vi "circular buffer test.vi"() -> ()   [LabVIEW 2010]
panel:
  out "size(s) 4":i32
  out "size(s) 3":i32
  out "size(s) 2":i32
  in  "stop":bool
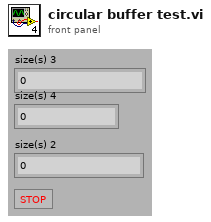
[diagram p1: front panel]
types:
  T1 = enum16{"CreateBuffer", "WriteBytes", "WriteByte", "AvailableMemory", "OccupiedMemory", "CheckBytes", "ReadBytes"}
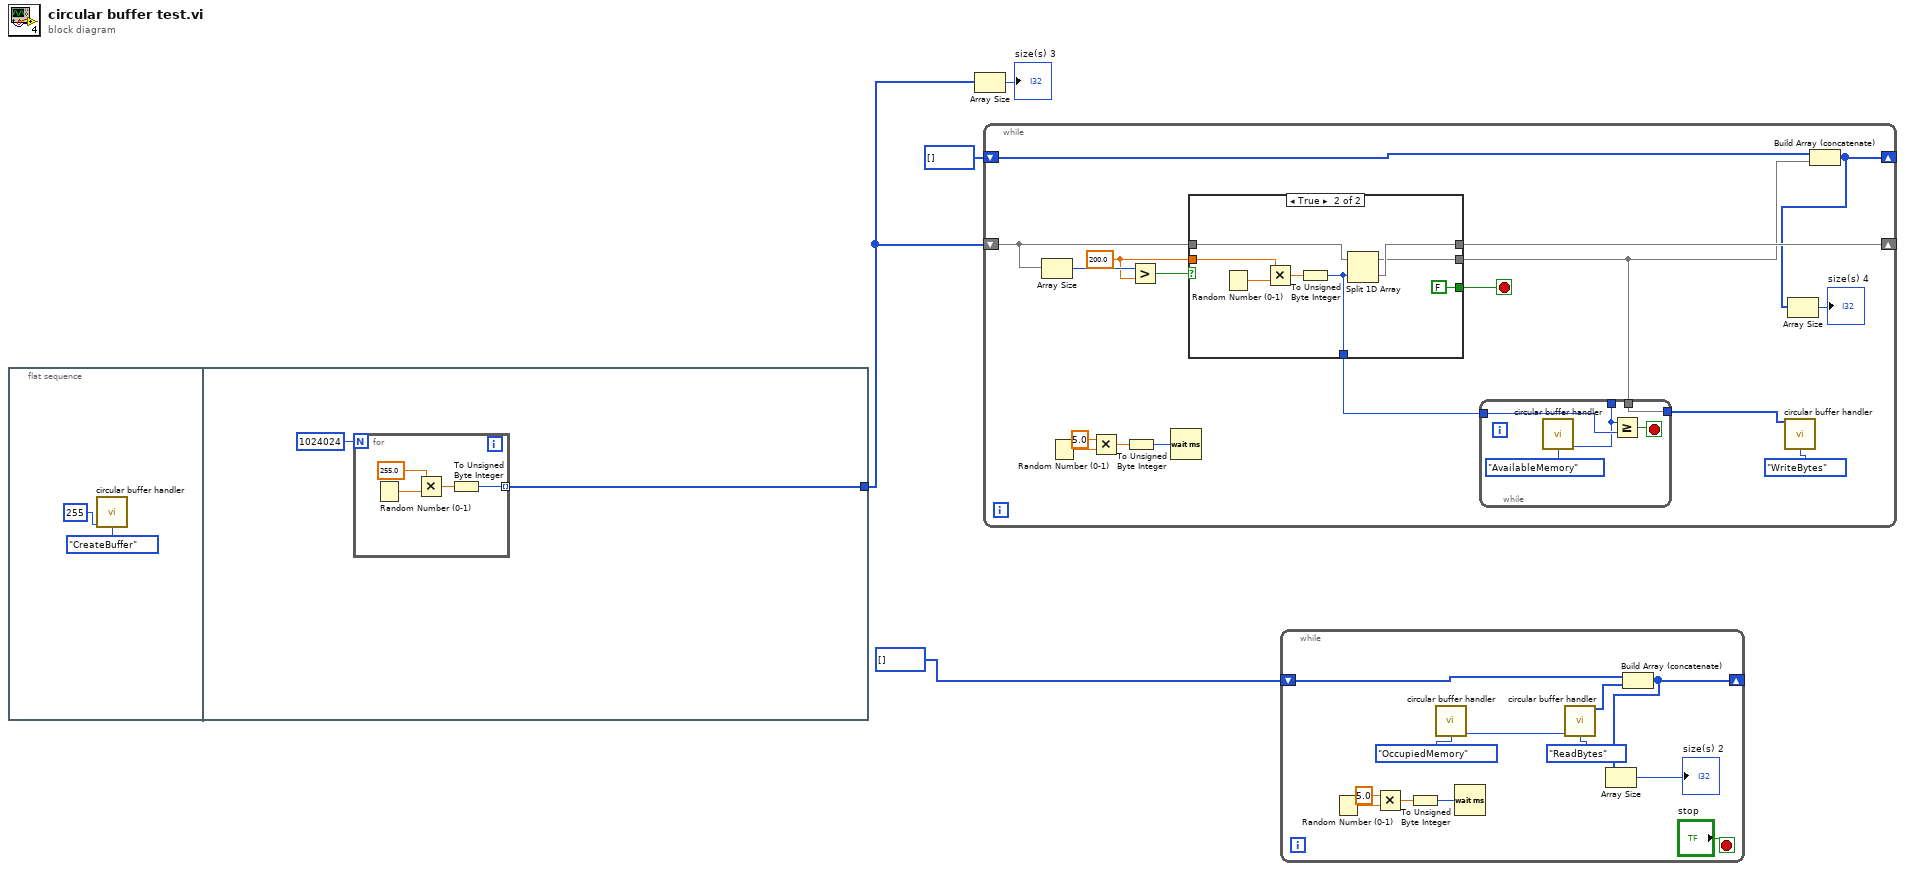
[diagram p0: block diagram]
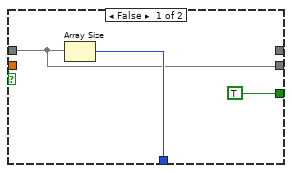
[diagram p2: hidden frame]
diagram:
  n1 = flat-sequence {
    tunnel: [w7] -> w2
    frame #0 {
      n2 = call "circular buffer handler.vi"("NumberOfBytes"=255 ("ByteToWrite"), "Enum"=T1."CreateBuffer") -> ()  [unwired: 11 in, 3 out]
    }
    frame #1 {
      n3 = for {
        N: 1024024 -> [_]
        tunnel: [w9] -> w7 mode=indexing
        n4 = Random Number (0-1)() -> (number: 0 to 1=w12:dbl)
        n5 = Multiply(x=255.0, y=w12) -> (x*y=w10:dbl)
        n6 = To Unsigned Byte Integer(number=w10) -> (unsigned 8bit integer=w9:u8)
      }
    }
  }
  n7 = Array Size(array=w2) -> (size(s)=→"size(s) 3":i32)
  n8 = while {
    shift-right: [w28] -> _
    shift-left: w2 -> [w26]
    shift-right: [w13] -> _
    shift-left: u8[] [] -> [w21]
    stop <- w22 stop-if-true
    w23 = 200.0 ("x")
    n9 = Array Size(array=w26) -> (size(s)=w25:i32)
    n10 = Random Number (0-1)() -> (number: 0 to 1=w18:dbl)
    n11 = Multiply(x=5.0, y=w18) -> (x*y=w17:dbl)
    n12 = To Unsigned Byte Integer(number=w17) -> (unsigned 8bit integer=w16:u8)
    n13 = Greater?(x=w25, y=w23) -> (0:w24:bool)
    n14 = Wait (ms)(milliseconds to wait=w16) -> ()  [unwired: 1 out]
    n15 = case shown="True" w24 {
      tunnel: w26 -> [w30 w38]
      tunnel: [_ w37] -> w28
      tunnel: [w32 w36] -> w27
      tunnel: w23 -> [_ w35]
      tunnel: [TRUE FALSE] -> w22
      tunnel: [w30 w33] -> w20
      frame False {
        n16 = Array Size(array=w30) -> (size(s)=w32:i32)
      }
      frame True {
        n17 = Random Number (0-1)() -> (number: 0 to 1=w39:dbl)
        n18 = Multiply(x=w35, y=w39) -> (x*y=w40:dbl)
        n19 = To Unsigned Byte Integer(number=w40) -> (unsigned 8bit integer=w36:u8)
        n20 = Split 1D Array(array=w38, index=w36) -> (first subarray=w33:u8[], second subarray=w37:u8[])
      }
    }
    n21 = while {
      tunnel: w27 -> [w45]
      tunnel: [w42] -> _
      tunnel: [w41] -> w19
      tunnel: w20 -> [w41]
      stop <- w44 stop-if-true
      n22 = call "circular buffer handler.vi"("Enum"=T1."AvailableMemory") -> ("Output"=w42:i32)  [unwired: 12 in, 2 out]
      n23 = Greater Or Equal?(x=w42, y=w45) -> (x >= y?=w44:bool)
    }
    n24 = call "circular buffer handler.vi"("StreamToWrite"=w19, "Enum"=T1."WriteBytes") -> ()  [unwired: 11 in, 3 out]
    n25 = Build Array (concatenate)(w21, w20) -> (w13:u8[])
    n26 = Array Size(array=w13) -> (size(s)=→"size(s) 4":i32)
  }
  n27 = while {
    shift-right: [w46] -> _
    shift-left: u8[] [] -> [w53]
    stop <- "stop" stop-if-true
    n28 = Random Number (0-1)() -> (number: 0 to 1=w48:dbl)
    n29 = Multiply(x=5.0, y=w48) -> (x*y=w49:dbl)
    n30 = To Unsigned Byte Integer(number=w49) -> (unsigned 8bit integer=w50:u8)
    n31 = call "circular buffer handler.vi"("Enum"=T1."OccupiedMemory") -> ("Output"=w52:i32)  [unwired: 12 in, 2 out]
    n32 = Wait (ms)(milliseconds to wait=w50) -> ()  [unwired: 1 out]
    n33 = call "circular buffer handler.vi"("NumberOfBytes"=w52, "Enum"=T1."ReadBytes") -> ("OutputBytes"=w54:u8[])  [unwired: 11 in, 2 out]
    n34 = Build Array (concatenate)(w53, w54) -> (w46:u8[])
    n35 = Array Size(array=w46) -> (size(s)=→"size(s) 2":i32)
  }
